vi "ViewAnalysisResults.vi"(7 "LabVIEW Web Service Request":refnum<class "Web Request.lvclass">) -> (3 "Data":T1)   [LabVIEW 2019]
uses:
  <vilib>/wsapi/Web Request.lvclass
  Private Content/ParameterData.ctl
  Private Content/WebServicesData.ctl
panel:
  # "Use the Web Service Request input terminal to call the VIs on the Web Services palette. Do not remove it from the connector pane unless you don't need access to the palette."
  # "Each additional control wired to the connector pane will be available as an input in the URL. To include an indicator in terminal-mode output (the default setting), it must also be wired to the connector pane."
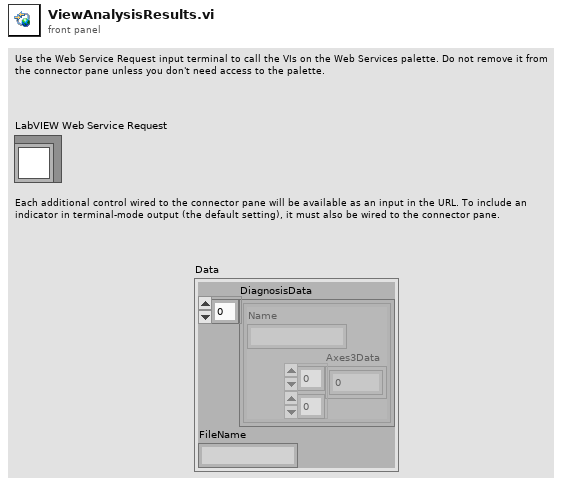
[diagram p1: front panel]
types:
  T1 = typedef "WebServicesData.ctl" = cluster{"DiagnosisData":T2[], "FileName":string}
  T2 = typedef "ParameterData.ctl" = cluster{"Name":string, "Axes3Data":dbl[][]}
  T3 = enum16{"open", "open or create", "create or replace", "create", "open (read-only)"}
  T4 = enum16{"open", "replace", "create", "open or create", "replace or create", "replace or create with confirmation"}
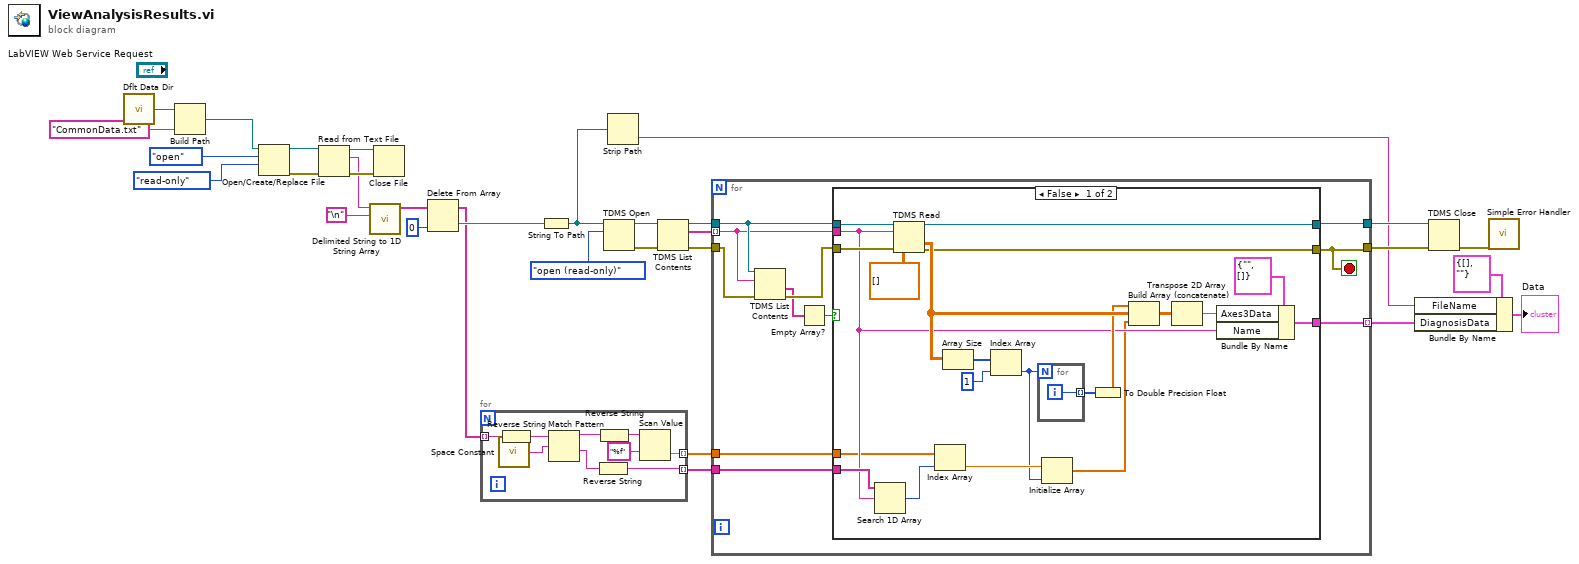
[diagram p0: block diagram]
diagram:
  n1 = call <vilib>:"Dflt Data Dir.vi"() -> ("App:Default Data Directory"=w31:path)
  n2 = Build Path(base path=w31, name or relative path="CommonData.txt") -> (appended path=w29:path)
  n3 = Open/Create/Replace File(file path (use dialog)=w29, operation (0:open)=T4."open", access (0:read/write)=enum16{"read/write", "read-only", "write-only"}."read-only") -> (refnum out=w26:refnum<file>, error out=w25:errorcluster)  [unwired: 3 in, 1 out]
  n4 = Read from Text File(file (use dialog)=w26, error in=w25) -> (refnum out=w24:refnum<file>, text=w13:string, error out=w23:errorcluster)  [unwired: 2 in, 1 out]
  n5 = call <vilib>:"Delimited String to 1D String Array.vi"("delimiter"="\n", "delimited string"=w13) -> ("string array"=w11:string[])  [unwired: 9 in]
  n6 = Close File(refnum=w24, error in=w23) -> ()  [unwired: 2 out]
  n7 = Delete From Array(array=w11, index=0) -> (deleted portion=w9:string, array with subset deleted=w8:string[])  [unwired: 1 in]
  n8 = for {
    tunnel: w8 -> [w40] mode=indexing
    tunnel: [w35] -> w6 mode=indexing
    tunnel: [w32] -> w7 mode=indexing
    n9 = call <vilib>:"Space Constant.vi"() -> ("String"=w38:string)
    n10 = Reverse String(1:w40) -> (0:w39:string)
    n11 = Match Pattern(string=w39, regular expression=w38) -> (before substring=w37:string, after substring=w36:string)  [unwired: 1 in, 2 out]
    n12 = Reverse String(1:w36) -> (0:w35:string)
    n13 = Reverse String(1:w37) -> (0:w34:string)
    n14 = Scan Value(string=w34, format string="%f") -> (value=w32:dbl)  [unwired: 1 in, 1 out]
  }
  n15 = String To Path(string=w9) -> (path=w5:path)
  n16 = TDMS Open(10:T3."open (read-only)" ("operation (0:open)"), 11:w5) -> (0:w20:errorcluster, 3:w21:refnum<k34>)  [unwired: 5 in]
  n17 = Strip Path(path=w5) -> (name=w3:string)  [unwired: 1 out]
  n18 = TDMS List Contents(4:w20, 7:w21) -> (0:w17:errorcluster, 2:w18:string[], 3:w19:refnum<k34>)  [unwired: 1 in, 1 out]
  n19 = for {
    tunnel: w19 -> [w46]
    tunnel: w18 -> [w45] mode=indexing
    tunnel: w17 -> [w48]
    tunnel: [w51] -> w16
    tunnel: [w49] -> w15
    tunnel: [w50] -> w4 mode=indexing
    tunnel: w7 -> [w42]
    tunnel: w6 -> [w41]
    stop <- w49 stop-if-true
    n20 = TDMS List Contents(4:w48, 6:w45, 7:w46) -> (0:w47:errorcluster, 1:w43:string[])  [unwired: 2 out]
    n21 = Empty Array?(array=w43) -> (empty?=w44:bool)
    n22 = case shown="False" w44 {
      tunnel: w46 -> [w72 w75]
      tunnel: w47 -> [w71 w74]
      tunnel: [w69 w75] -> w51
      tunnel: w45 -> [w58 _]
      tunnel: [w68 _] -> w50
      tunnel: [w61 w74] -> w49
      tunnel: w42 -> [w57 _]
      tunnel: w41 -> [w59 _]
      frame False {
        n23 = Search 1D Array(1D array=w59, element=w58) -> (index of element=w56:i32)  [unwired: 1 in]
        n24 = TDMS Read(0:w72, 5:w58, 11:w71, 12:dbl[][] []) -> (4:w69:refnum<k34>, 10:w63:dbl[][], 15:w61:errorcluster)  [unwired: 4 in, 3 out]
        n25 = Index Array(array=w57, index=w56) -> (element=w55:dbl)
        n26 = Array Size(array=w63) -> (size(s)=w67:i32[])
        n27 = Index Array(array=w67, index=1) -> (element=w54:i32)
        n28 = for {
          N: w54 -> [_]
          tunnel: [w73] -> w65 mode=indexing
          i -> [w73]
        }
        n29 = Initialize Array(w55, w54) -> (w53:dbl[])
        n30 = To Double Precision Float(number=w65) -> (double precision float=w62:dbl[])
        n31 = Build Array (concatenate)(w62, w63, w53) -> (w64:dbl[][])
        n32 = Transpose 2D Array(2D array=w64) -> (transposed array=w60:dbl[][])
        n33 = Bundle By Name(cluster=T2 {"Name"="", "Axes3Data"=[]} ("Parameter"), "Axes3Data"=w60, "Name"=w58) -> (w68:T2)
      }
      frame True {
      }
    }
  }
  n34 = Bundle By Name(cluster=T1 {"DiagnosisData"=[], "FileName"=""} ("WebServicesData"), "FileName"=w3, "DiagnosisData"=w4) -> (→"Data":T1)
  n35 = TDMS Close(8:w15, 11:w16) -> (0:w14:errorcluster)  [unwired: 1 out]
  n36 = call <vilib>:"Simple Error Handler.vi"("error in (no error)"=w14) -> ()  [unwired: 4 in, 5 out]
